vi "Close.vi"(8 "error in":errorcluster, 11 "UserEventHandler in":refnum<class "UserEventHandler.lvclass">) -> (0 "error out":errorcluster, 3 "UserEventHandler out":refnum<class "UserEventHandler.lvclass">)   [LabVIEW 2020, in "hse-logger.lvlib" / "UserEventHandler.lvclass"]
doc: "Destroys the user event. This method should be called when the ``Logger`` gets closed or the handler is removed from the ``Logger``.\n\n____\nHAMPEL SOFTWARE ENGINEERING v2.0.6 (2021-04-15 11:38)"
uses:
  UserEventHandler.lvclass
  UserEventHandler.lvclass/UserEventHandler.ctl
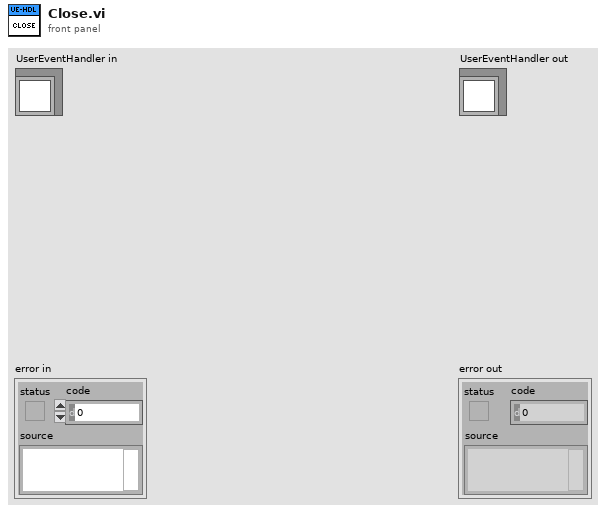
[diagram p1: front panel]
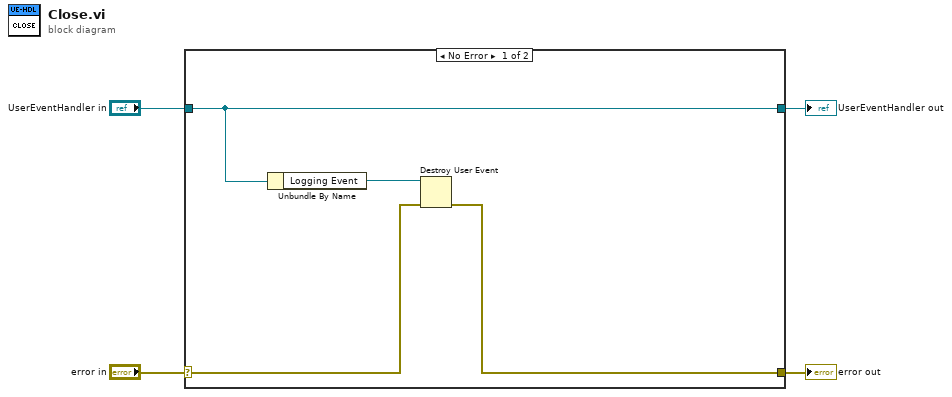
[diagram p0: block diagram]
diagram:
  n1 = case shown="No Error" "error in" {
    selector: "error in" -> [w6 w10]
    tunnel: [w5 w10] -> w3
    tunnel: [w8 w9] -> w1
    tunnel: "UserEventHandler in" -> [w8 w9]
    frame No Error {
      n2 = Unbundle By Name(w8) -> ("Logging Event"=w7:refnum<user-event>)
      n3 = Destroy User Event(user event=w7, error in=w6) -> (error out=w5:errorcluster)
    }
    frame Error {
    }
  }
  "error out" <- w3
  "UserEventHandler out" <- w1
